vi "Player Info.vi"(11 "Cross in":refnum<class "Cross.lvclass">) -> (1 "Victory Speech":string, 2 "Name":string, 3 "Cross out":refnum<class "Cross.lvclass">)   [LabVIEW 2015, in "Cross.lvclass"]
uses:
  Cross.lvclass
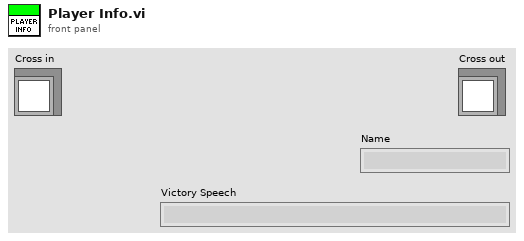
[diagram p1: front panel]
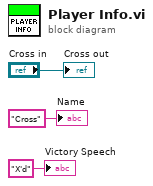
[diagram p0: block diagram]
diagram:
  "Cross out" <- "Cross in"
  "Name" <- "Cross"
  "Victory Speech" <- "X'd"
